vi "Add Tx Generic Command Section and Channels.vi"(8 "error in":errorcluster, 11 "Tx generic ref in":T1 format="%.0x") -> (0 "error out":errorcluster, 1 "Tx generic command channel refs":T1[](array[typedef]) format="%.0x", 2 "Tx generic status section ref out":T1 format="%.0x", 3 "Tx generic ref out":T1 format="%.0x")   [LabVIEW 2020, in "AIM ARINC 664 Scripting.lvlib"]
uses:
  AIM ARINC 664 Scripting.lvlib
  <vilib>/NI VeriStand/Custom Device API/Custom Device API.lvlib
  <vilib>/NI VeriStand/Custom Device API/Custom Device Channel Type.ctl
  <vilib>/NI VeriStand/Custom Device API/Custom Device Channel.ctl
  Constants.vi
  <vilib>/NI VeriStand/Custom Device API/Custom Device Item Ref.ctl
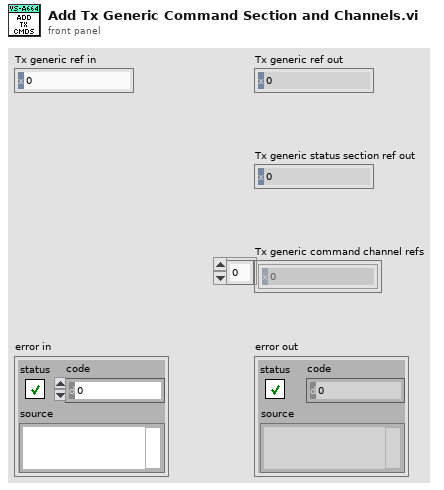
[diagram p1: front panel]
types:
  T1 = typedef "Custom Device API.lvlib/Custom Device Item Ref.ctl" = u64
  T2 = typedef "Custom Device API.lvlib/Custom Device Channel.ctl" = cluster{"Type":T3, "Units":string, "Default Value":dbl, "Faultable":bool, "Scalable":bool}
  T3 = typedef "Custom Device API.lvlib/Custom Device Channel Type.ctl" = enum16{"Input", "Output"}
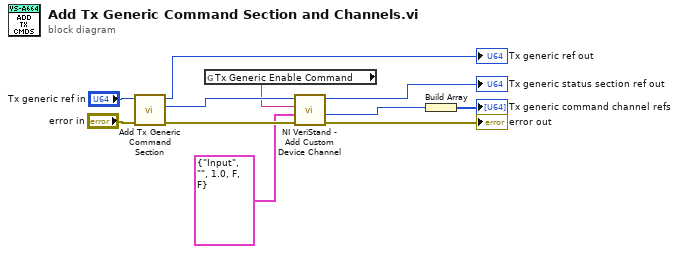
[diagram p0: block diagram]
diagram:
  n1 = call "Add Tx Generic Command Section.vi"("error in"="error in", "Tx generic ref in"="Tx generic ref in") -> ("error out"=w5:errorcluster, "Tx generic command section ref out"=w6:T1, "Tx generic ref out"=→"Tx generic ref out":T1)  [unwired: 7 in]
  n2 = global read "Constants.vi" "Tx Generic Enable Command"() -> (w1:string)
  n3 = call <vilib>:"NI VeriStand - Add Custom Device Channel.vi"("error in (no error)"=w5, "Channel"=T2 {"Type"=enum."Input", "Units"="", "Default Value"=1.0, "Faultable"=FALSE, "Scalable"=FALSE}, "Channel Name"=w1, "Parent Ref in"=w6) -> ("error out"=→"error out":errorcluster, "Channel Ref"=w8:T1, "Parent Ref out"=→"Tx generic status section ref out":T1)  [unwired: 4 in, 1 out]
  n4 = Build Array(w8) -> (→"Tx generic command channel refs":T1[])
